vi "Get Name.vi"(8 "error in (no error)":errorcluster, 11 "RFFE RegReadExt Command in":refnum<class "RFFE RegReadExt Command.lvclass">) -> (0 "error out":errorcluster, 2 "Name":string, 3 "RFFE RegReadExt Command out":refnum<class "RFFE RegReadExt Command.lvclass">)   [LabVIEW 2018, in "MIPI RFFE API.lvlib" / "RFFE RegReadExt Command.lvclass"]
uses:
  RFFE RegReadExt Command.lvclass
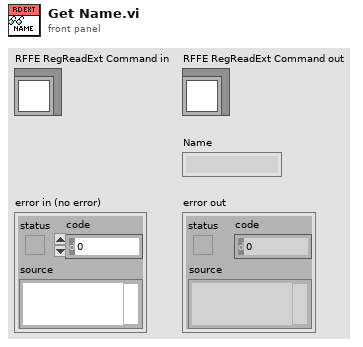
[diagram p1: front panel]
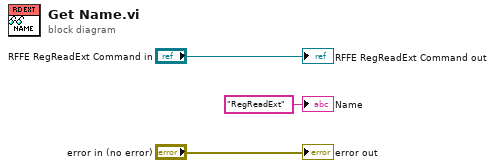
[diagram p0: block diagram]
diagram:
  "error out" <- "error in (no error)"
  "RFFE RegReadExt Command out" <- "RFFE RegReadExt Command in"
  "Name" <- "RegReadExt" ("Name")
